vi "from string 2.0.vi"(8 "error in":errorcluster, 10 "data in":string, 11 "Shared Memory configuration in":refnum<class "Shared Memory configuration.lvclass">) -> (0 "error out":errorcluster, 2 "remaining data":string, 3 "Shared Memory configuration out":refnum<class "Shared Memory configuration.lvclass">)   [LabVIEW 2014, in "Shared Memory configuration.lvclass"]
uses:
  Shared Memory configuration.lvclass
  <vilib>/NI/Tag Bus Module Framework/channel/TBM channel.lvclass
  Line.ctl
  Shared Memory configuration.lvclass/Shared Memory configuration.ctl
  <vilib>/NI/Configuration Framework/serializable configuration/NISE_CEF_serializable configuration.lvclass
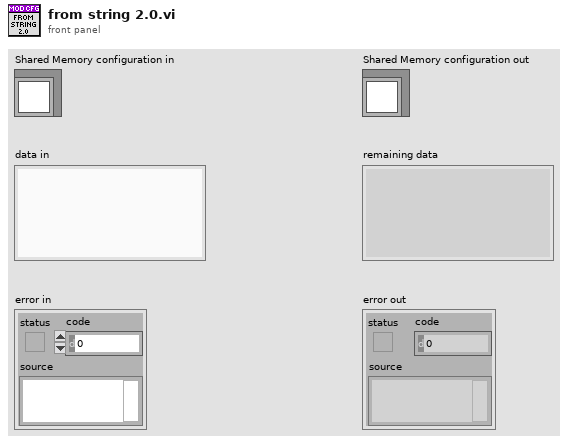
[diagram p1: front panel]
types:
  T1 = typedef "Shared Memory configuration.lvclass/Line.ctl" = cluster{"channel":refnum<class "TBM channel.lvclass">}
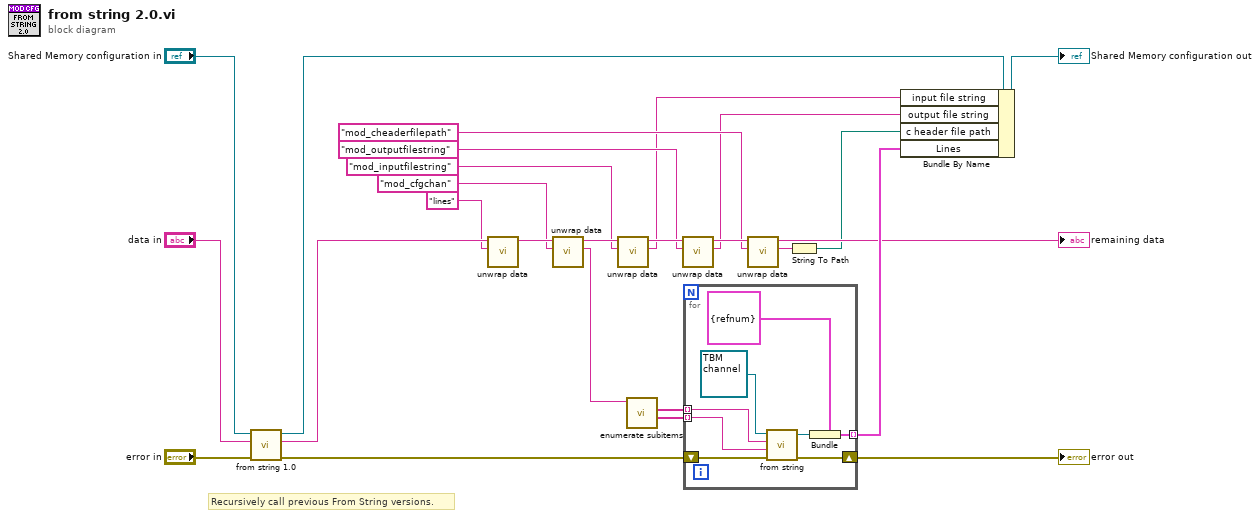
[diagram p0: block diagram]
diagram:
  # "Recursively call previous From String versions."
  n1 = call "from string 1.0.vi"("error in"="error in", "data in"="data in", "Shared Memory configuration in"="Shared Memory configuration in") -> ("error out"=w12:errorcluster, "remaining data"=w8:string, "Shared Memory configuration out"=w10:refnum<class "Shared Memory configuration.lvclass">)  [unwired: 6 in]
  n2 = call <vilib>:"unwrap data.vi"("identifier"="lines" ("additional identifier"), "data to unwrap"=w8) -> ("remaining string"=w23:string)  [unwired: 8 in, 1 out]
  n3 = call <vilib>:"unwrap data.vi"("identifier"="mod_cfgchan", "data to unwrap"=w23) -> ("unwrapped data"=w20:string, "remaining string"=w7:string)  [unwired: 8 in]
  n4 = call <vilib>:"unwrap data.vi"("identifier"="mod_inputfilestring", "data to unwrap"=w7) -> ("unwrapped data"=w2:string, "remaining string"=w18:string)  [unwired: 8 in]
  n5 = call <vilib>:"enumerate subitems.vi"("data to enumerate"=w20) -> ("associated data"=w21:string[], "discovered subitems"=w22:string[])  [unwired: 8 in, 1 out]
  n6 = call <vilib>:"unwrap data.vi"("identifier"="mod_outputfilestring", "data to unwrap"=w18) -> ("unwrapped data"=w1:string, "remaining string"=w17:string)  [unwired: 8 in]
  n7 = for {
    shift-right: [w34] -> w11
    shift-left: w12 -> [w33]
    tunnel: w22 -> [w32] mode=indexing
    tunnel: w21 -> [w31] mode=indexing
    tunnel: [w27] -> w19 mode=indexing
    n8 = call-dynamic "from string.vi"("error in"=w33, "channel data"=w31, "identifier"=w32, "channel in"=refnum<class "TBM channel.lvclass"> refnum) -> ("error out"=w34:errorcluster, "channel out"=w28:refnum<class "TBM channel.lvclass">)  [unwired: 6 in]
    n9 = Bundle(cluster=T1 {"channel"=refnum} ("Line"), "channel"=w28) -> (w27:T1)
  }
  "error out" <- w11
  n10 = call <vilib>:"unwrap data.vi"("identifier"="mod_cheaderfilepath", "data to unwrap"=w17) -> ("unwrapped data"=w4:string, "remaining string"=→"remaining data":string)  [unwired: 8 in]
  n11 = String To Path(string=w4) -> (path=w3:path)
  n12 = Bundle By Name(cluster=w10, "input file string"=w2, "output file string"=w1, "c header file path"=w3, "Lines"=w19) -> (→"Shared Memory configuration out":refnum<class "Shared Memory configuration.lvclass">)
